vi "Attempt Backlog Transmission.vi"(8 "error in (no error)":errorcluster, 11 "SessionHandler in":refnum<class "SessionHandler.lvclass">) -> (0 "error out":errorcluster, 3 "SessionHandler out":refnum<class "SessionHandler.lvclass">)   [LabVIEW 2017, in "Network Sink.lvlib" / "SessionHandler.lvclass"]
uses:
  <vilib>/gpm_packages/@cs/event-logger/Source/Network Sink/SessionHandler/SessionHandler.lvclass
  <vilib>/gpm_packages/@cs/event-logger/Source/Network Sink/SessionHandler/SessionHandler.lvclass/SessionHandler.ctl
  <vilib>/gpm_packages/@cs/event-logger/Source/Composed Log/Types/Log Level.ctl
  <vilib>/gpm_packages/@cs/event-logger/Source/Composed Log/Composed Log.lvlib
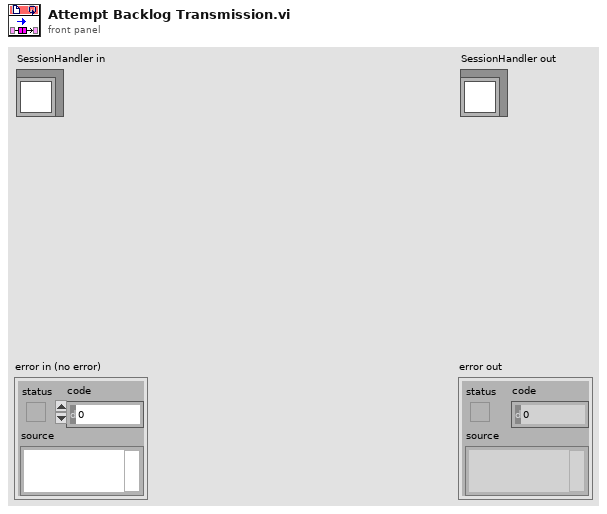
[diagram p1: front panel]
types:
  T1 = typedef "Composed Log.lvlib/Log Level.ctl" = enum16{"Debug", "Info", "Warning", "Error", "Critical"}
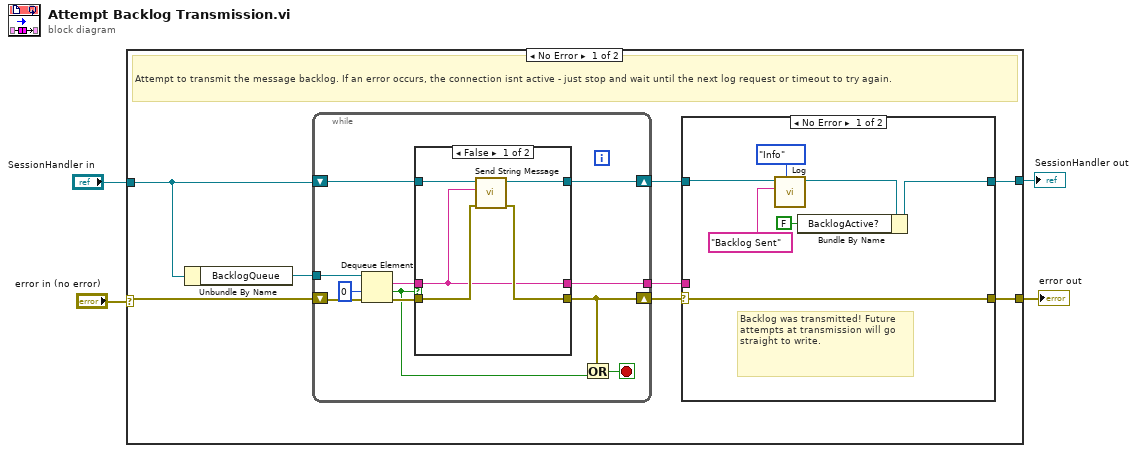
[diagram p0: block diagram]
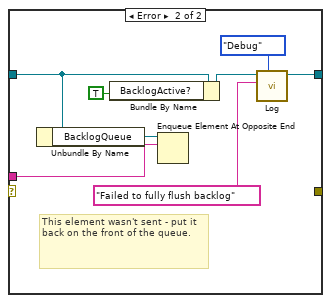
[diagram p2: hidden frame]
diagram:
  n1 = case shown="No Error" "error in (no error)" {
    selector: "error in (no error)" -> [w5 w47]
    tunnel: [w9 w47] -> w3
    tunnel: [w7 w46] -> w1
    tunnel: "SessionHandler in" -> [w11 w46]
    frame No Error {
      # "Attempt to transmit the message backlog. If an error occurs, the connection isnt active - just stop and wait until the next log request or timeout to try again."
      n2 = Unbundle By Name(w11) -> ("BacklogQueue"=w12:refnum<queue>)
      n3 = while {
        shift-right: [w34] -> w8
        shift-left: w11 -> [w35]
        tunnel: w12 -> [w38]
        shift-right: [w29] -> w10
        shift-left: w5 -> [w36]
        tunnel: [w28] -> w6
        stop <- w31 stop-if-true
        n4 = Dequeue Element(queue=w38, timeout in ms (-1)=0, error in (no error)=w36) -> (element=w33:string, timed out?=w30:bool, error out=w32:errorcluster)  [unwired: 1 out]
        n5 = case shown="False" w30 {
          tunnel: w35 -> [w43 w45]
          tunnel: [w42 w45] -> w34
          tunnel: w33 -> [w39 _]
          tunnel: w32 -> [w41 w44]
          tunnel: [w40 w44] -> w29
          tunnel: [w39 _] -> w28
          frame False {
            n6 = call <vilib>:"Send String Message.vi"("error in (no error)"=w41, "Data To Write"=w39, "SessionHandler in"=w43) -> ("error out"=w40:errorcluster, "SessionHandler out"=w42:refnum<class "SessionHandler.lvclass">)  [unwired: 7 in]
          }
          frame True {
          }
        }
        n7 = Or(x=w29, y=w30) -> (x .or. y?=w31:bool)
      }
      n8 = case shown="No Error" w10 {
        selector: w10 -> [w19 _]
        tunnel: [w19 _] -> w9
        tunnel: w8 -> [w15 w27]
        tunnel: [w18 w22] -> w7
        tunnel: w6 -> [_ w25]
        frame No Error {
          # "Backlog was transmitted! Future attempts at transmission will go straight to write."
          n9 = call <vilib>:"Log.vi"("Event Level"=Log_Level."Info", "Data To Log"="Backlog Sent", "SessionHandler in"=w15) -> ("SessionHandler out"=w14:refnum<class "SessionHandler.lvclass">)  [unwired: 7 in, 1 out]
          n10 = Bundle By Name(cluster=w14, "BacklogActive?"=FALSE) -> (w18:refnum<class "SessionHandler.lvclass">)
        }
        frame Error {
          # "This element wasn't sent - put it back on the front of the queue."
          n11 = Unbundle By Name(w27) -> ("BacklogQueue"=w26:refnum<queue>)
          n12 = Bundle By Name(cluster=w27, "BacklogActive?"=TRUE) -> (w23:refnum<class "SessionHandler.lvclass">)
          n13 = Enqueue Element At Opposite End(queue=w26, element=w25) -> ()  [unwired: 2 in, 3 out]
          n14 = call <vilib>:"Log.vi"("Event Level"=Log_Level."Debug", "Data To Log"="Failed to fully flush backlog", "SessionHandler in"=w23) -> ("SessionHandler out"=w22:refnum<class "SessionHandler.lvclass">)  [unwired: 7 in, 1 out]
        }
      }
    }
    frame Error {
    }
  }
  "error out" <- w3
  "SessionHandler out" <- w1
